vi "testConnection.vi"(8 "error in (no error)":errorcluster, 11 "db_File":path=path "C:/Users/YuanYuan/Desktop/Labview Data/Database") -> (0 "error out":errorcluster)   [LabVIEW 2014]
uses:
  <vilib>/addons/database/Connection.llb/DB Tools Open Connec (String).vi
  <vilib>/addons/database/NI_Database_API.lvlib
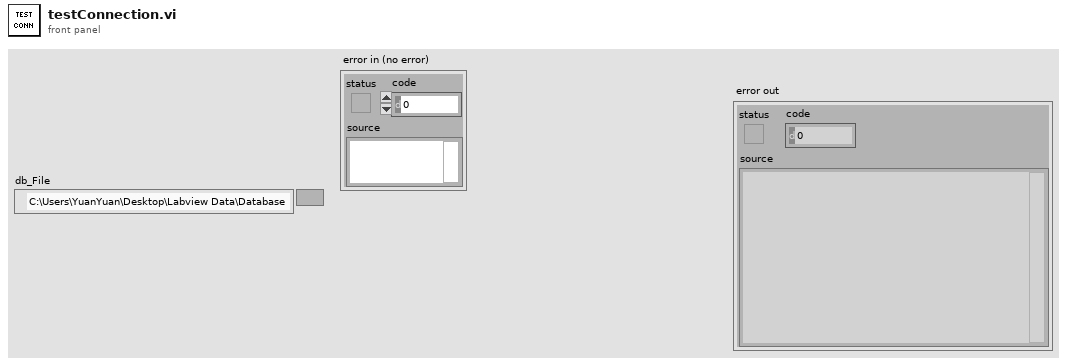
[diagram p1: front panel]
types:
  T1 = typedef "NI_Database_API.lvlib/Conn ObjectReference.ctl" = refnum<k1>
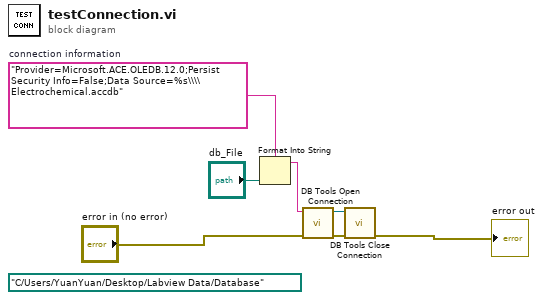
[diagram p0: block diagram]
diagram:
  (unwired) path "C:/Users/YuanYuan/Desktop/Labview Data/Database" ("path")
  w7 = "Provider=Microsoft.ACE.OLEDB.12.0;Persist Security Info=False;Data Source=%s\\\\Electrochemical.accdb"  # connection information
  n1 = Format Into String(format string=w7, "db_File") -> (resulting string=w5:string)  [unwired: 2 in, 1 out]
  n2 = call-poly <vilib>:"DB Tools Open Connection.vi"("error in (no error)"="error in (no error)", "connection information"=w5) -> ("error out"=w2:errorcluster, "connection reference"=w3:T1)  [unwired: 6 in]
  n3 = call <vilib>:"DB Tools Close Connection.vi"("error in (no error)"=w2, "connection reference"=w3) -> ("error out"=→"error out":errorcluster)  [unwired: 5 in]
